vi "AlliGator Preview ROI File.vi"(8 "Error In":errorcluster, 9 "Destination Image":string="Source Image", 11 "File Path":path) -> (0 "Error Out":errorcluster, 1 "Phasor Plot Image":bool, 3 "# ROIs Loaded":i32)   [LabVIEW 2021, in "AlliGator ROIs.lvlib"]
doc: "Returns information on ROIs stored in the file."
uses:
  Image/ROI XML Format.ctl
  Image/Image Control ROI Description.ctl
  Image/Image Control Multiple ROIs Description.ctl
  Image/Image Control ROI Description v2.ctl
  Image/Named ROI Description.ctl
  Image/Image Control Multiple ROIs Description v2.ctl
  8ad5fe3a-6877-4cbc-8fef-4c072b65eab6.vi
  454e6171-cdfd-4cb8-a5e3-eaa046060a80.vi
  <vilib>/JDP Science/JSONtext/JSON text to Variant.vi
  <vilib>/Utility/error.llb/Error Cluster From Error Code.vi
  <vilib>/JDP Science/JSONtext/LVClass Serializer/JSONtext LVClass Serializer.lvclass
  <vilib>/ErrorRing/Error Ring.xnode
  AlliGator ROIs.lvlib
  Image/Image.lvlib
  Files/Files.lvlib
  Time/Time.lvlib
panel:
  out "Time (s)":dbl
  # "see the AlliGator License on the block diagram (Ctrl+E or Window:Show Block Diagram)"
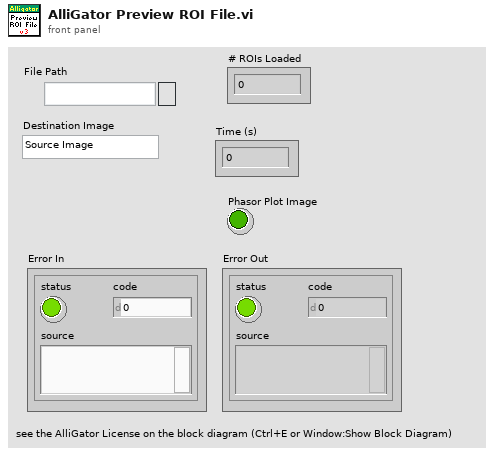
[diagram p1: front panel]
types:
  T1 = typedef "Image.lvlib/ROI XML Format.ctl" = enum16{"Single ROI v1", "Multiple ROIs v1", "Single ROI v2", "Multiple ROIs v2", "Single ROI v3", "Multiple ROIs v3", "Exit"}
  T2 = typedef "Image.lvlib/Image Control ROI Description.ctl" = cluster{"Image Control Label":string, "ROI Descriptor":T3}
  T3 = typedef "ROI Descriptor" = cluster{"Global Rectangle":i32[], "Contours":cluster{"ID":enum32{"External", "Internal"}, "Type":u32, "Coordinates":i32[]}[]}
  T4 = typedef "Image.lvlib/Image Control Multiple ROIs Description.ctl" = cluster{"Image Control Label":string, "ROI Descriptors":T3[]}
  T5 = typedef "Image.lvlib/Image Control ROI Description v2.ctl" = cluster{"Image Control Label":string, "Named ROI Description":T6}
  T6 = typedef "Image.lvlib/Named ROI Description.ctl" = cluster{"ROI Descriptor":T3, "ROI Name":string, "Overlay Color":u32}
  T7 = typedef "Image.lvlib/Image Control Multiple ROIs Description v2.ctl" = cluster{"Image Control Label":string, "Named ROI Descriptions":T6[]}
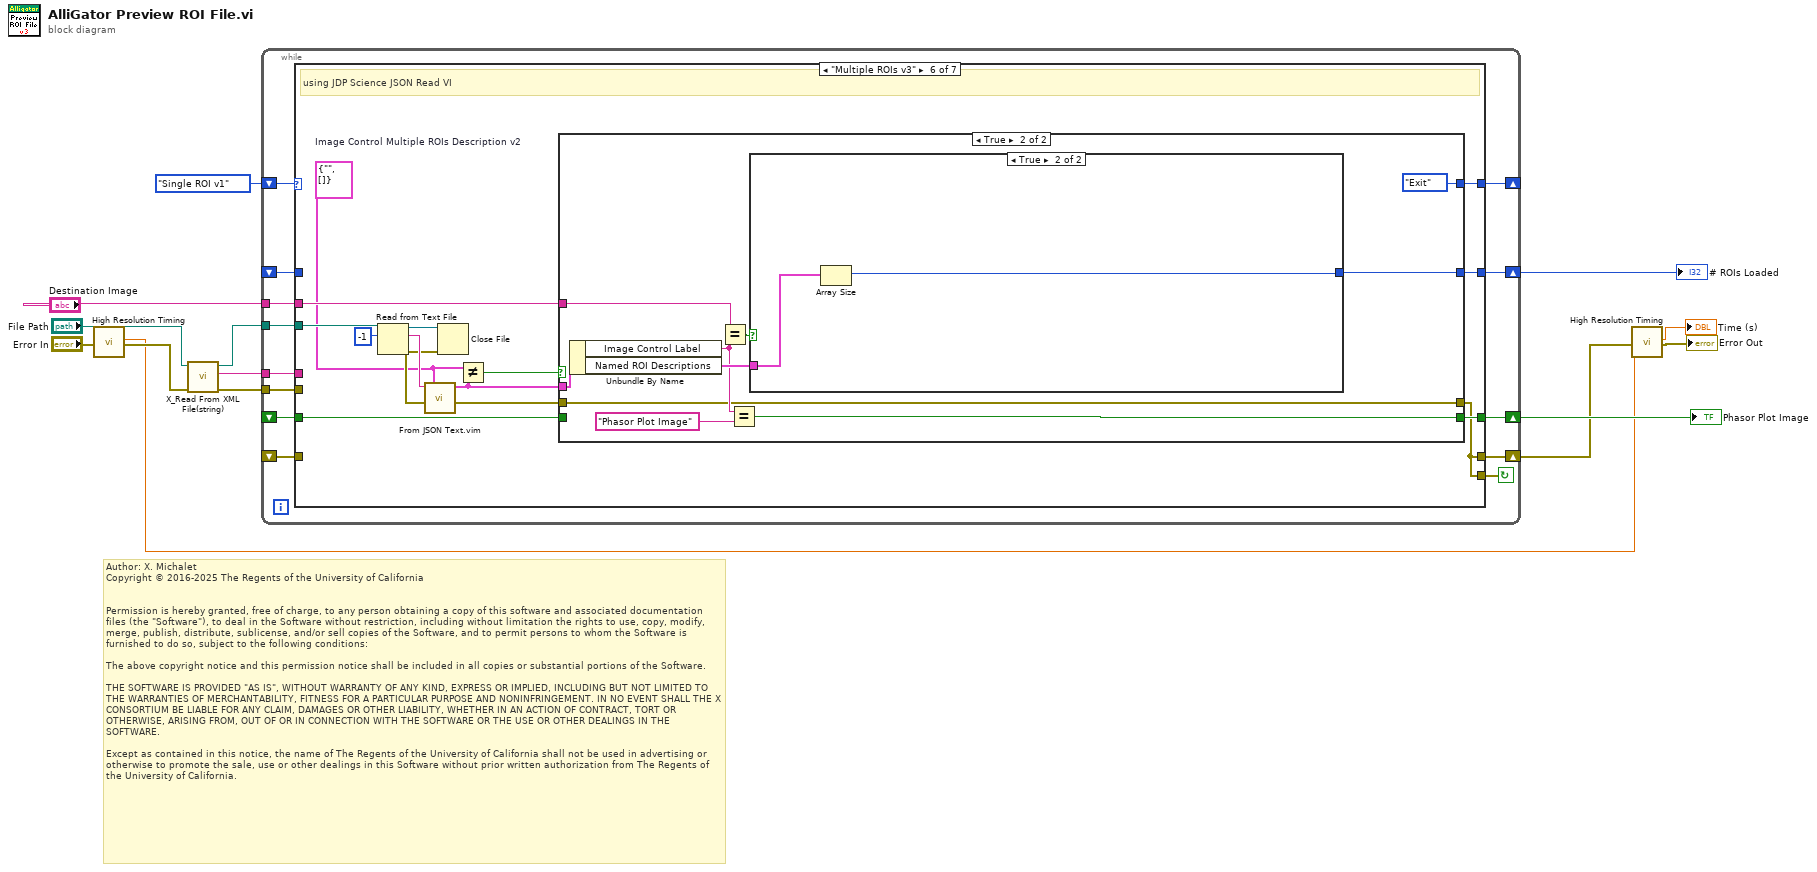
[diagram p0: block diagram]
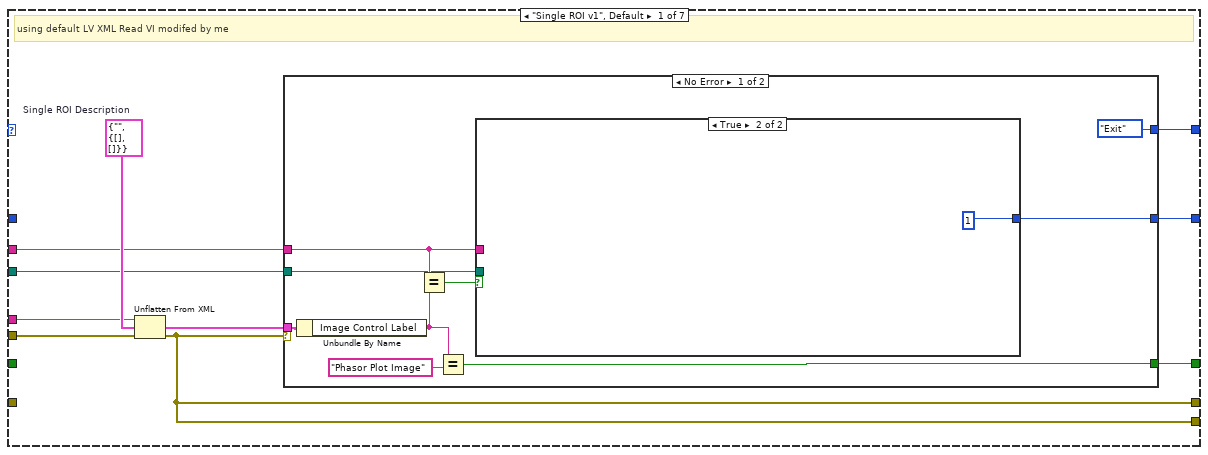
[diagram p2: hidden frame]
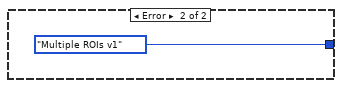
[diagram p4: hidden frame]
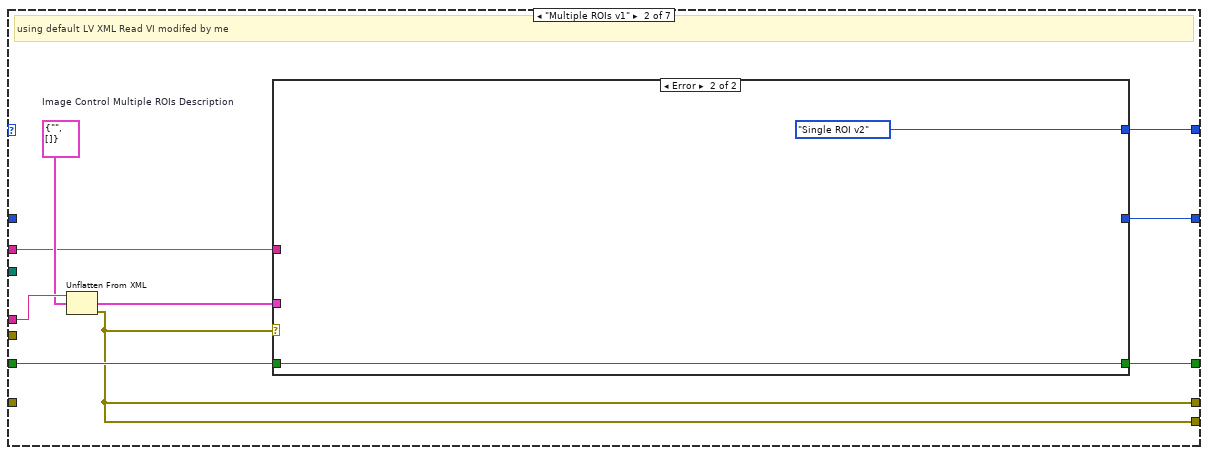
[diagram p5: hidden frame]
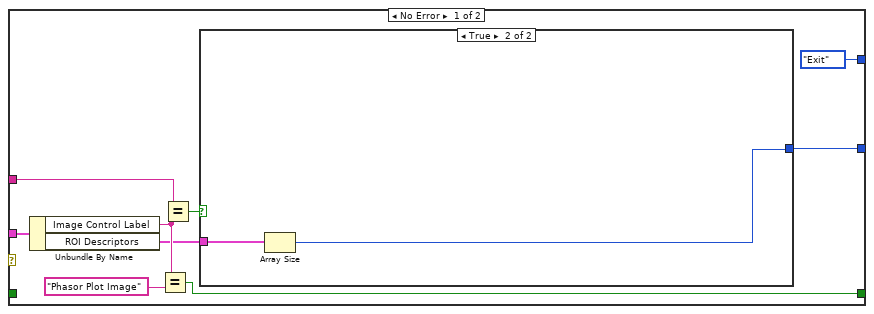
[diagram p6: hidden frame]
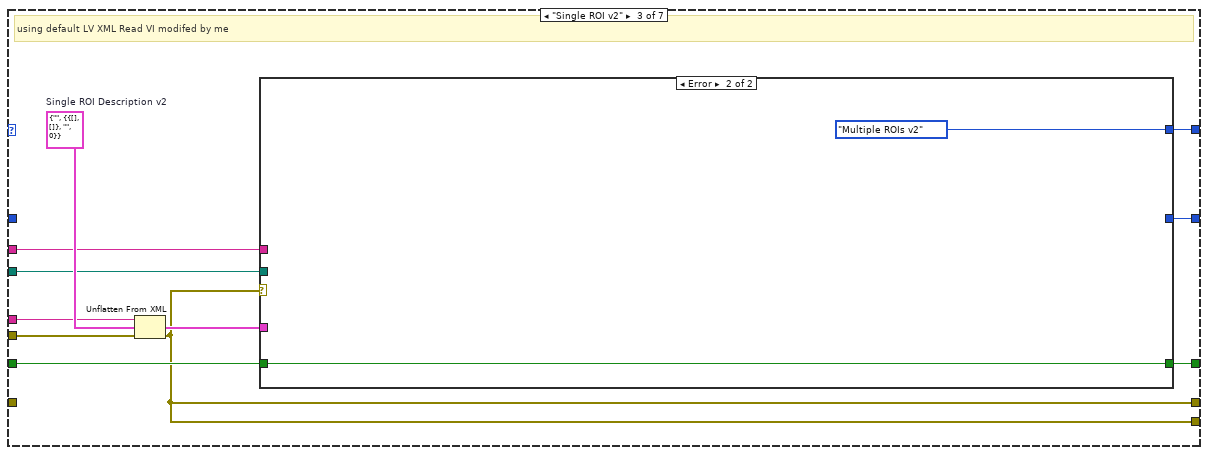
[diagram p8: hidden frame]
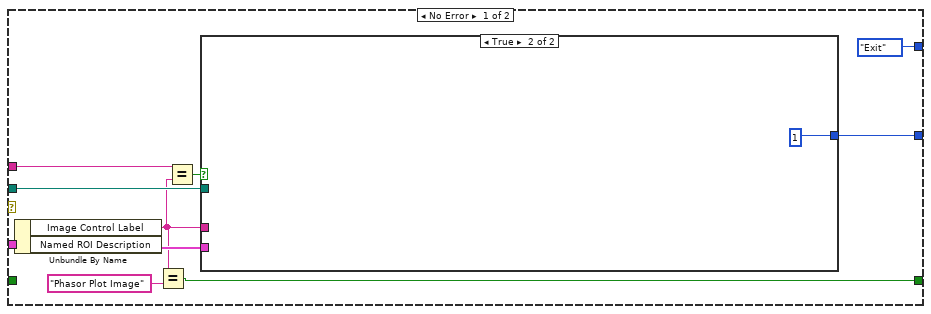
[diagram p9: hidden frame]
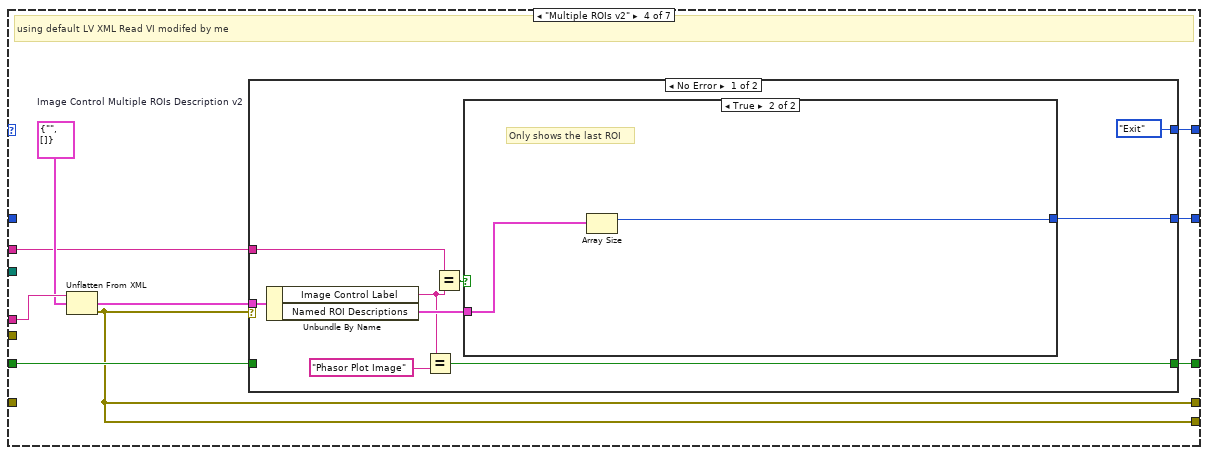
[diagram p11: hidden frame]
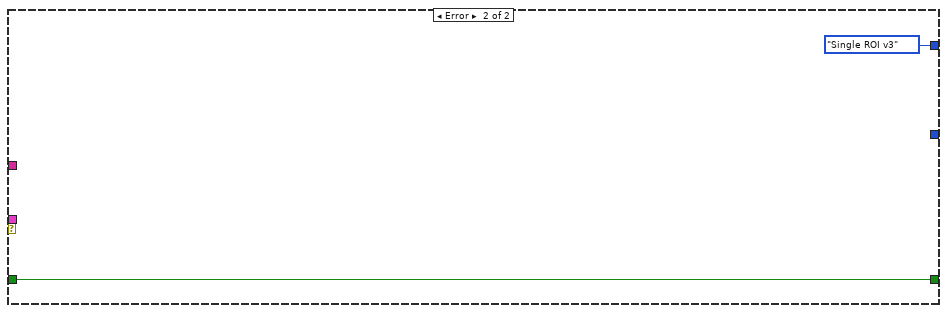
[diagram p13: hidden frame]
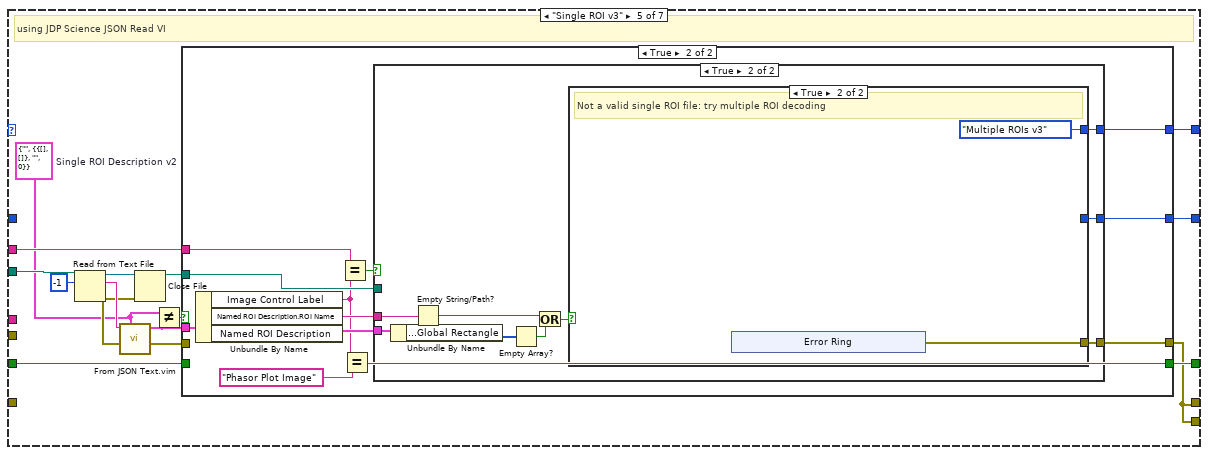
[diagram p14: hidden frame]
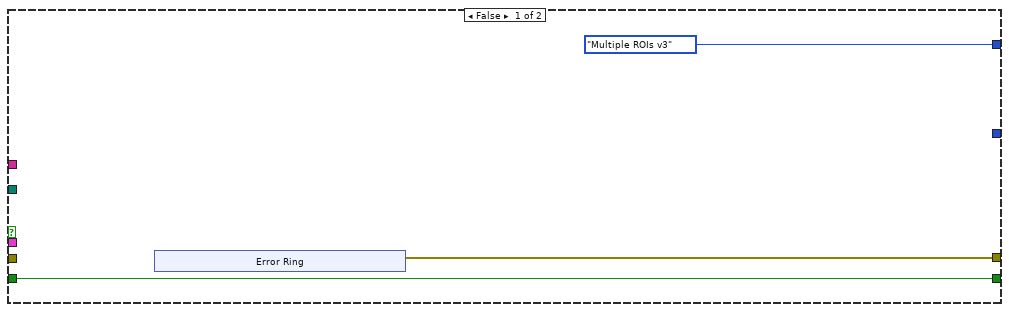
[diagram p15: hidden frame]
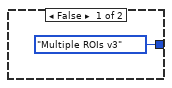
[diagram p16: hidden frame]
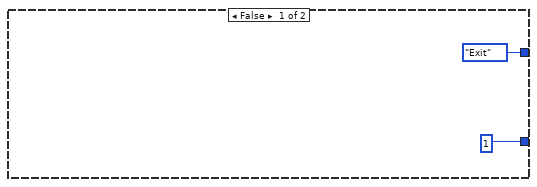
[diagram p17: hidden frame]
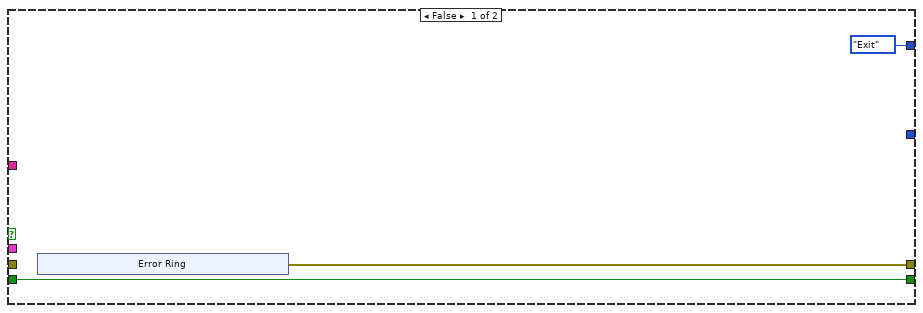
[diagram p18: hidden frame]
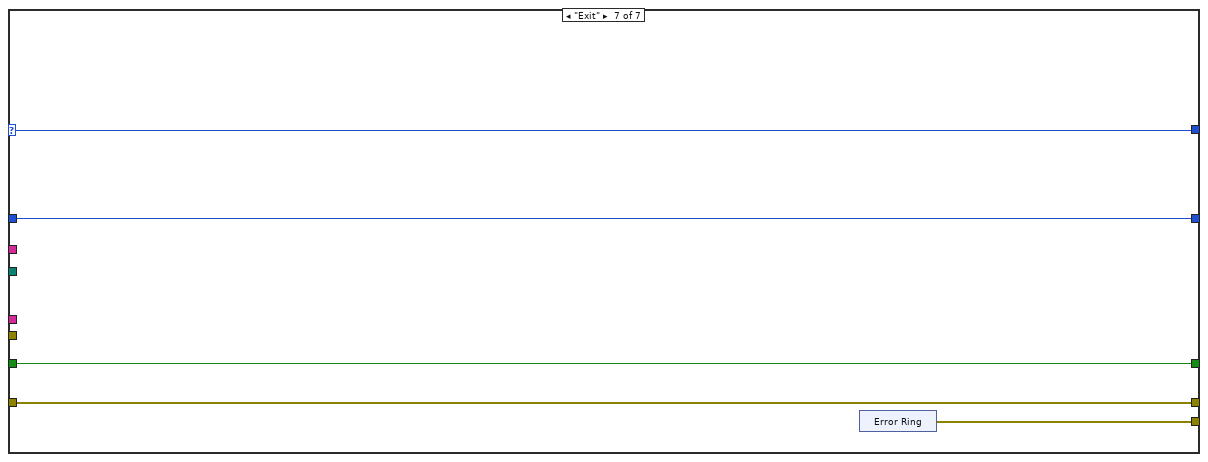
[diagram p20: hidden frame]
diagram:
  # "Author: X. Michalet\nCopyright © 2016-2025 The Regents of the University of California\n \n\nPermission is hereby granted, free of charge, to any person obtaining a copy of this software and associated documentation files (the \"Software\"), to deal in the Software without restriction, including without limitation the rights to use, copy, modify, merge, publish, distribute, sublicense, and/or sell copies of the Software, and to permit persons to whom the Software is furnished to do so, subject to the following conditions:\n\nThe above copyright notice and this permission notice shall be included in all copies or substantial portions of the Software.\n\nTHE SOFTWARE IS PROVIDED \"AS IS\", WITHOUT WARRANTY OF ANY KIND, EXPRESS OR IMPLIED, INCLUDING BUT NOT LIMITED TO THE WARRANTIES OF MERCHANTABILITY, FITNESS FOR A PARTICULAR PURPOSE AND NONINFRINGEMENT. IN NO EVENT SHALL THE X CONSORTIUM BE LIABLE FOR ANY CLAIM, DAMAGES OR OTHER LIABILITY, WHETHER IN AN ACTION OF CONTRACT, TORT OR OTHERWISE, ARISING FROM, OUT OF OR IN CONNECTION WITH THE SOFTWARE OR THE USE OR OTHER DEALINGS IN THE SOFTWARE.\n\nExcept as contained in this notice, the name of The Regents of the University of California shall not be used in advertising or otherwise to promote the sale, use or other dealings in this Software without prior written authorization from The Regents of the University of California."
  n1 = call "High Resolution Timing.vi"("Error In"="Error In") -> ("elapsed (relative) seconds"=w7:dbl, "Error Out"=w8:errorcluster)  [unwired: 16 in, 1 out]
  n2 = call "X_Read From XML File(string).vi"("error in (no error)"=w8, "XML File Path"="File Path") -> ("error out"=w6:errorcluster, "XML Elements"=w4:string, "XML File Path(duplicate)"=w5:path)  [unwired: 7 in]
  n3 = while {
    tunnel: w5 -> [w26]
    tunnel: w4 -> [w25]
    shift-right: [w20] -> _
    shift-left: ROI_XML_Format."Single ROI v1" -> [w22]
    shift-right: [w23] -> w3
    shift-left: _ -> [w19]
    shift-right: [w24] -> w14
    shift-left: _ -> [w18]
    tunnel: "Destination Image" -> [w17]
    tunnel: w6 -> [w27]
    shift-right: [w16] -> w1
    shift-left: _ -> [w15]
    stop <- w21 continue-if-true
    n4 = case shown="\"Multiple ROIs v3\"" w22 {
      selector: w22 -> [_ _ _ _ _ _ w208]
      tunnel: w27 -> [w36 _ w80 _ _ _ _]
      tunnel: w26 -> [w34 _ w78 _ w129 w181 _]
      tunnel: w25 -> [w33 w57 w77 w103 _ _ _]
      tunnel: [w32 w52 w76 w98 w132 w182 w206] -> w24
      tunnel: [w31 w56 w75 w102 w131 w184 w204] -> w23
      tunnel: [w28 w49 w71 w95 w120 w170 w207] -> w21
      tunnel: [w30 w53 w74 w99 w130 w183 w208] -> w20
      tunnel: w19 -> [_ _ _ _ _ _ w204]
      tunnel: w18 -> [_ w51 w73 w97 w127 w180 w206]
      tunnel: w17 -> [w29 w50 w72 w96 w126 w179 _]
      tunnel: [w28 w49 w71 w95 w120 w170 w205] -> w16
      tunnel: w15 -> [_ _ _ _ _ _ w205]
      frame "Single ROI v1", Default {
        w37 = T2 {"Image Control Label"="", "ROI Descriptor"={"Global Rectangle"=[], "Contours"=[]}}  # Single ROI Description
        # "using default LV XML Read VI modifed by me"
        n5 = Unflatten From XML(xml string=w33, type=w37, error in (no error)=w36) -> (value=w35:T2, error out=w28:errorcluster)
        n6 = case shown="No Error" w28 {
          tunnel: w35 -> [w46 _]
          tunnel: w29 -> [w45 _]
          tunnel: w34 -> [w44 _]
          tunnel: [w38 _] -> w32
          tunnel: [w43 _] -> w31
          tunnel: [ROI_XML_Format."Exit" ROI_XML_Format."Multiple ROIs v1"] -> w30
          frame No Error {
            n7 = Unbundle By Name(w46) -> ("Image Control Label"=w41:string)
            n8 = Equal?(x=w45, y=w41) -> (x = y?=w42:bool)
            n9 = Equal?(x=w41, y="Phasor Plot Image") -> (x = y?=w38:bool)
            n10 = case shown="True" w42 {
              tunnel: w44 -> [_ _]
              tunnel: w45 -> [_ _]
              tunnel: [_ 1 ("value")] -> w43
              frame False {
              }
              frame True {
              }
            }
          }
          frame Error {
          }
        }
      }
      frame "Multiple ROIs v1" {
        w55 = T4 {"Image Control Label"="", "ROI Descriptors"=[]}  # Image Control Multiple ROIs Description
        # "using default LV XML Read VI modifed by me"
        n11 = Unflatten From XML(xml string=w57, type=w55) -> (value=w54:T4, error out=w49:errorcluster)  [unwired: 1 in]
        n12 = case shown="Error" w49 {
          tunnel: w54 -> [w66 _]
          tunnel: [w64 _] -> w56
          tunnel: [ROI_XML_Format."Exit" ROI_XML_Format."Single ROI v2"] -> w53
          tunnel: [w60 w69] -> w52
          tunnel: w51 -> [_ w69]
          tunnel: w50 -> [w59 _]
          frame No Error {
            n13 = Unbundle By Name(w66) -> ("Image Control Label"=w61:string, "ROI Descriptors"=w58:T3[])
            n14 = Equal?(x=w61, y="Phasor Plot Image") -> (x = y?=w60:bool)
            n15 = Equal?(x=w59, y=w61) -> (x = y?=w65:bool)
            n16 = case shown="True" w65 {
              tunnel: w58 -> [_ w68]
              tunnel: [_ w67] -> w64
              frame False {
              }
              frame True {
                n17 = Array Size(array=w68) -> (size(s)=w67:i32)
              }
            }
          }
          frame Error {
          }
        }
      }
      frame "Single ROI v2" {
        w81 = T5 {"Image Control Label"="", "Named ROI Description"={"ROI Descriptor"={"Global Rectangle"=[], "Contours"=[]}, "ROI Name"="", "Overlay Color"=0}}  # Single ROI Description v2
        # "using default LV XML Read VI modifed by me"
        n18 = Unflatten From XML(xml string=w77, type=w81, error in (no error)=w80) -> (value=w79:T5, error out=w71:errorcluster)
        n19 = case shown="Error" w71 {
          tunnel: w79 -> [w91 _]
          tunnel: w78 -> [w90 _]
          tunnel: [w82 w93] -> w76
          tunnel: [w89 _] -> w75
          tunnel: [ROI_XML_Format."Exit" ROI_XML_Format."Multiple ROIs v2"] -> w74
          tunnel: w73 -> [_ w93]
          tunnel: w72 -> [w84 _]
          frame No Error {
            n20 = Unbundle By Name(w91) -> ("Image Control Label"=w86:string, "Named ROI Description"=w87:T6)
            n21 = Equal?(x=w86, y="Phasor Plot Image") -> (x = y?=w82:bool)
            n22 = Equal?(x=w84, y=w86) -> (x = y?=w88:bool)
            n23 = case shown="True" w88 {
              tunnel: w87 -> [_ _]
              tunnel: w90 -> [_ _]
              tunnel: w86 -> [_ _]
              tunnel: [_ 1 ("value")] -> w89
              frame False {
              }
              frame True {
              }
            }
          }
          frame Error {
          }
        }
      }
      frame "Multiple ROIs v2" {
        w101 = T7 {"Image Control Label"="", "Named ROI Descriptions"=[]}  # Image Control Multiple ROIs Description v2
        # "using default LV XML Read VI modifed by me"
        n24 = Unflatten From XML(xml string=w103, type=w101) -> (value=w100:T7, error out=w95:errorcluster)  [unwired: 1 in]
        n25 = case shown="No Error" w95 {
          tunnel: w100 -> [w112 _]
          tunnel: [w109 _] -> w102
          tunnel: [ROI_XML_Format."Exit" ROI_XML_Format."Single ROI v3"] -> w99
          tunnel: [w105 w115] -> w98
          tunnel: w97 -> [_ w115]
          tunnel: w96 -> [w104 _]
          frame No Error {
            n26 = Unbundle By Name(w112) -> ("Image Control Label"=w106:string, "Named ROI Descriptions"=w110:T6[])
            n27 = Equal?(x=w106, y="Phasor Plot Image") -> (x = y?=w105:bool)
            n28 = Equal?(x=w104, y=w106) -> (x = y?=w111:bool)
            n29 = case shown="True" w111 {
              tunnel: w110 -> [_ w114]
              tunnel: [_ w113] -> w109
              frame False {
              }
              frame True {
                # "Only shows the last ROI"
                n30 = Array Size(array=w114) -> (size(s)=w113:i32)
              }
            }
          }
          frame Error {
          }
        }
      }
      frame "Single ROI v3" {
        w119 = T5 {"Image Control Label"="", "Named ROI Description"={"ROI Descriptor"={"Global Rectangle"=[], "Contours"=[]}, "ROI Name"="", "Overlay Color"=0}}  # Single ROI Description v2
        # "using JDP Science JSON Read VI"
        n31 = Read from Text File(file (use dialog)=w129, count=-1) -> (refnum out=w123:refnum<file>, text=w124:string, error out=w122:errorcluster)  [unwired: 2 in, 1 out]
        n32 = call "From JSON Text.vim"("Data Type and Default Value"=w119, "error in (no error)"=w122, "JSON"=w124) -> ("error out"=w121:errorcluster, "Data out"=w118:T5)  [unwired: 7 in]
        n33 = Close File(refnum=w123, error in=w122) -> (path=w128:path)  [unwired: 1 out]
        n34 = Not Equal?(x=w119, y=w118) -> (x != y?=w117:bool)
        n35 = case shown="True" w117 {
          tunnel: w118 -> [_ w151]
          tunnel: w128 -> [_ w150]
          tunnel: [w134 w141] -> w132
          tunnel: [_ w149] -> w131
          tunnel: [ROI_XML_Format."Multiple ROIs v3" w145] -> w130
          tunnel: w127 -> [w134 _]
          tunnel: w126 -> [_ w144]
          tunnel: [w133 w140] -> w120
          tunnel: w121 -> [_ _]
          frame False {
            n36 = xnode "Error Ring"() -> ("error out"=w133:errorcluster)
          }
          frame True {
            n37 = Unbundle By Name(w151) -> ("Image Control Label"=w143:string, "Named ROI Description.ROI Name"=w146:string, "Named ROI Description"=w147:T6)
            n38 = Equal?(x=w144, y=w143) -> (x = y?=w148:bool)
            n39 = Equal?(x=w143, y="Phasor Plot Image") -> (x = y?=w141:bool)
            n40 = case shown="True" w148 {
              tunnel: w147 -> [_ w160]
              tunnel: w150 -> [_ _]
              tunnel: [_ w161] -> w149
              tunnel: w146 -> [_ w159]
              tunnel: [ROI_XML_Format."Multiple ROIs v3" w156] -> w145
              tunnel: [_ w153] -> w140
              frame False {
              }
              frame True {
                n41 = Unbundle By Name(w160) -> ("ROI Descriptor.Global Rectangle"=w158:i32[])
                n42 = Empty String/Path?(string/path=w159) -> (empty?=w155:bool)
                n43 = Empty Array?(array=w158) -> (empty?=w154:bool)
                n44 = Or(x=w155, y=w154) -> (x .or. y?=w157:bool)
                n45 = case shown="True" w157 {
                  tunnel: [1 ("value") _] -> w161
                  tunnel: [ROI_XML_Format."Exit" ROI_XML_Format."Multiple ROIs v3"] -> w156
                  tunnel: [_ w164] -> w153
                  frame False {
                  }
                  frame True {
                    # "Not a valid single ROI file: try multiple ROI decoding"
                    n46 = xnode "Error Ring"() -> ("error out"=w164:errorcluster)
                  }
                }
              }
            }
          }
        }
      }
      frame "Multiple ROIs v3" {
        w173 = T7 {"Image Control Label"="", "Named ROI Descriptions"=[]}  # Image Control Multiple ROIs Description v2
        # "using JDP Science JSON Read VI"
        n47 = Read from Text File(file (use dialog)=w181, count=-1) -> (refnum out=w175:refnum<file>, text=w177:string, error out=w176:errorcluster)  [unwired: 2 in, 1 out]
        n48 = call "From JSON Text.vim"("Data Type and Default Value"=w173, "error in (no error)"=w176, "JSON"=w177) -> ("error out"=w174:errorcluster, "Data out"=w172:T7)  [unwired: 7 in]
        n49 = Close File(refnum=w175, error in=w176) -> ()  [unwired: 2 out]
        n50 = Not Equal?(x=w173, y=w172) -> (x != y?=w171:bool)
        n51 = case shown="True" w171 {
          tunnel: w172 -> [_ w201]
          tunnel: [_ w198] -> w184
          tunnel: [ROI_XML_Format."Exit" ROI_XML_Format."Exit"] -> w183
          tunnel: [w186 w194] -> w182
          tunnel: w180 -> [w186 _]
          tunnel: w179 -> [_ w193]
          tunnel: w174 -> [_ w192]
          tunnel: [w185 w192] -> w170
          frame False {
            n52 = xnode "Error Ring"() -> ("error out"=w185:errorcluster)
          }
          frame True {
            n53 = Unbundle By Name(w201) -> ("Image Control Label"=w195:string, "Named ROI Descriptions"=w199:T6[])
            n54 = Equal?(x=w193, y=w195) -> (x = y?=w200:bool)
            n55 = Equal?(x=w195, y="Phasor Plot Image") -> (x = y?=w194:bool)
            n56 = case shown="True" w200 {
              tunnel: w199 -> [_ w203]
              tunnel: [_ w202] -> w198
              frame False {
              }
              frame True {
                n57 = Array Size(array=w203) -> (size(s)=w202:i32)
              }
            }
          }
        }
      }
      frame "Exit" {
        n58 = xnode "Error Ring"() -> ("error out"=w207:errorcluster)
      }
    }
  }
  "Phasor Plot Image" <- w14
  "# ROIs Loaded" <- w3
  n59 = call "High Resolution Timing.vi"("relative seconds (NaN)"=w7, "Error In"=w1) -> ("elapsed (relative) seconds"=→"Time (s)":dbl, "Error Out"=→"Error Out":errorcluster)  [unwired: 15 in, 1 out]
